vi "Update Control from Metadata.vi"(6 "default_value":variant, 8 "error in":errorcluster, 9 "control name":string, 10 "parameter data":T1[](array[typedef]), 11 "vi refnum":refnum<vi>) -> (0 "error out":errorcluster)   [LabVIEW 2021, in "MeasurementClient Editor.lvlib"]
uses:
  MeasurementClient Editor.lvlib
  <vilib>/gRPC/Generated APIs/ni/measurementlink/measurement/v2/Measurement Service Client V2/RPC Messages/ni_measurementlink_measurement_v2_ConfigurationParameter.ctl
  <vilib>/gRPC/Generated APIs/ni/measurementlink/measurement/v2/Measurement Service Client V2/RPC Messages/google_protobuf_Field_Kind.ctl
  <vilib>/gRPC/Generated APIs/ni/measurementlink/measurement/v2/Measurement Service Client V2/RPC Messages/ni_measurementlink_measurement_v2_ConfigurationParameter_AnnotationsEntry.ctl
  <vilib>/Utility/miscctls.llb/LVPositionTypeDef.ctl
  <vilib>/gRPC/Generated APIs/ni/measurementlink/measurement/v2/Measurement Service Client V2/Measurement Service Client V2.lvlib
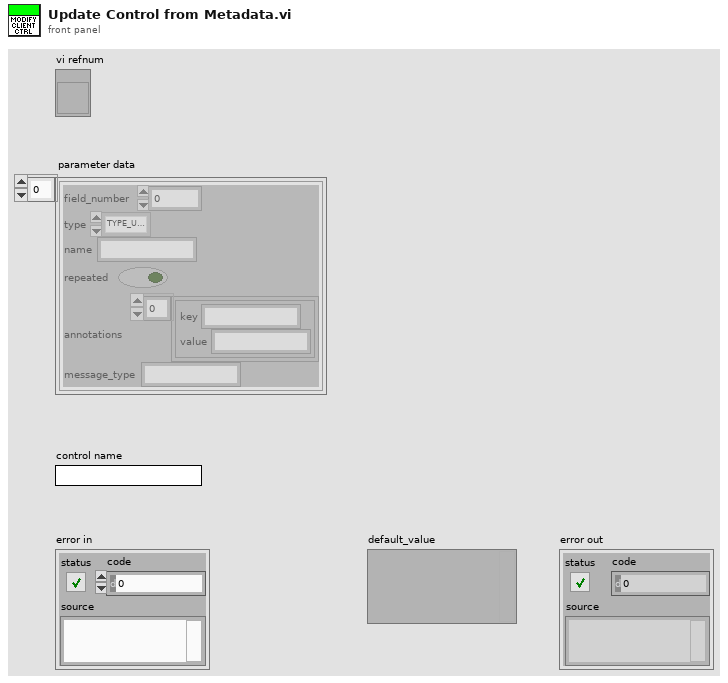
[diagram p1: front panel]
types:
  T1 = typedef "Measurement Service Client V2.lvlib/ni_measurementlink_measurement_v2_ConfigurationParameter.ctl" = cluster{"field_number":i32, "type":T2, "name":string, "repeated":bool, "annotations":T3[], "message_type":string}
  T2 = typedef "Measurement Service Client V2.lvlib/google_protobuf_Field_Kind.ctl" = enum32{"TYPE_UNKNOWN", "TYPE_DOUBLE", "TYPE_FLOAT", "TYPE_INT64", "TYPE_UINT64", "TYPE_INT32", "TYPE_FIXED64", "TYPE_FIXED32", "TYPE_BOOL", "TYPE_STRING", "TYPE_GROUP", "TYPE_MESSAGE", "TYPE_BYTES", "TYPE_UINT32", "TYPE_ENUM", "TYPE_SFIXED32", "TYPE_SFIXED64", "TYPE_SINT32", "TYPE_SINT64"}
  T3 = typedef "Measurement Service Client V2.lvlib/ni_measurementlink_measurement_v2_ConfigurationParameter_AnnotationsEntry.ctl" = cluster{"key":string, "value":string}
  T4 = typedef "LVPositionTypeDef.ctl" = cluster{"Left":i32, "Top":i32}
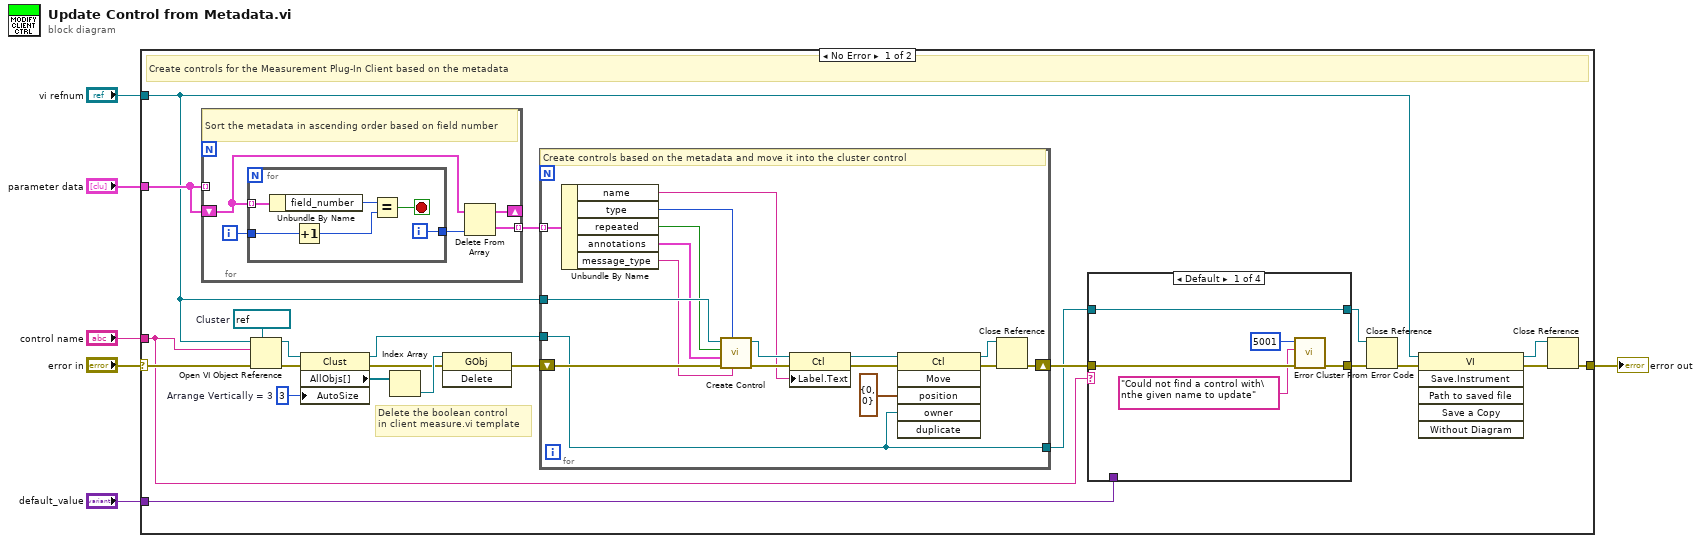
[diagram p0: block diagram]
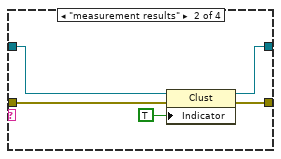
[diagram p2: hidden frame]
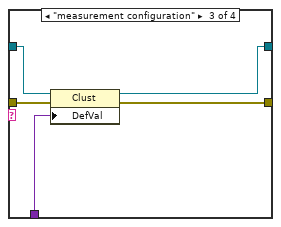
[diagram p3: hidden frame]
diagram:
  n1 = case shown="No Error" "error in" {
    selector: "error in" -> [w23 w75]
    tunnel: "control name" -> [w15 _]
    tunnel: "parameter data" -> [w13 _]
    tunnel: "vi refnum" -> [w10 _]
    tunnel: [w8 w75] -> w3
    tunnel: "default_value" -> [w7 _]
    frame No Error {
      w22 = u32 3  # Arrange Vertically = 3
      w29 = refnum<vi> refnum  # Cluster
      # "Delete the boolean control\nin client measure.vi template"
      # "Create controls for the Measurement Plug-In Client based on the metadata"
      n2 = for {
        shift-right: [w48] -> _
        shift-left: w13 -> [w49]
        tunnel: [w47] -> w14 mode=indexing
        tunnel: w13 -> [_] mode=indexing
        i -> [w51]
        # "Sort the metadata in ascending order based on field number"
        n3 = for {
          tunnel: w49 -> [w54] mode=indexing
          tunnel: w51 -> [w57]
          tunnel: [w53] -> w50
          i -> [w53]
          stop <- w52 stop-if-true
          n4 = Unbundle By Name(w54) -> ("field_number"=w56:i32)
          n5 = Increment(x=w57) -> (x+1=w55:i32)
          n6 = Equal?(x=w56, y=w55) -> (x = y?=w52:bool)
        }
        n7 = Delete From Array(array=w49, index=w50) -> (deleted portion=w47:T1, array with subset deleted=w48:T1[])  [unwired: 1 in]
      }
      n8 = Open VI Object Reference(7:w29, 8:w23, 10:w15, 11:w10) -> (0:w27:errorcluster, 3:w28:refnum<vi>)
      n9 = property class="Clust"(reference=w28, error in=w27, "AutoSize"=w22) -> (reference out=w19:refnum<vi>, error out=w24:errorcluster, "AllObjs[]"=w26:refnum<vi>[])
      n10 = Index Array(array=w26) -> (element=w25:refnum<vi>)  [unwired: 1 in]
      n11 = invoke class="GObj" method="Delete"(reference=w25, error in=w24) -> (error out=w21:errorcluster)  [unwired: 1 in, 2 out]
      n12 = for {
        shift-right: [w34] -> w20
        shift-left: w21 -> [w46]
        tunnel: w10 -> [w44]
        tunnel: w19 -> [w32]
        tunnel: [w32] -> w17
        tunnel: w14 -> [w30] mode=indexing
        # "Create controls based on the metadata and move it into the cluster control"
        n13 = Unbundle By Name(w30) -> ("name"=w38:string, "type"=w42:T2, "repeated"=w43:bool, "annotations"=w41:T3[], "message_type"=w40:string)
        n14 = call "Create Control.vi"("message_type"=w40, "type"=w42, "error in"=w46, "annotations"=w41, "is repeated?"=w43, "vi refnum"=w44) -> ("error out"=w45:errorcluster, "control ref"=w39:refnum<vi>)  [unwired: 4 in]
        n15 = property class="Ctl"(reference=w39, error in=w45, "Label.Text"=w38) -> (reference out=w37:refnum<vi>, error out=w36:errorcluster)
        n16 = invoke class="Ctl" method="Move"(reference=w37, error in=w36, "position"=T4 {"Left"=0, "Top"=0}, "owner"=w32) -> (reference out=w33:refnum<vi>, error out=w35:errorcluster)  [unwired: 2 in, 4 out]
        n17 = Close Reference(reference=w33, error in (no error)=w35) -> (error out=w34:errorcluster)
      }
      n18 = case shown="Default" w15 {
        tunnel: w20 -> [w62 w67 w72 w73]
        tunnel: [w60 w66 w71 w73] -> w18
        tunnel: w17 -> [w61 w65 w70 w74]
        tunnel: [w61 w64 w69 w74] -> w16
        tunnel: w7 -> [_ _ w68 _]
        frame Default {
          n19 = call <vilib>:"Error Cluster From Error Code.vi"("error in (no error)"=w62, "error message (\"\")"="Could not find a control with\nthe given name to update" ("error message (\"\")"), "error code (0)"=5001) -> ("error out"=w60:errorcluster)  [unwired: 6 in]
        }
        frame "measurement results" {
          n20 = property class="Clust"(reference=w65, error in=w67, "Indicator"=TRUE) -> (reference out=w64:refnum<vi>, error out=w66:errorcluster)
        }
        frame "measurement configuration" {
          n21 = property class="Clust"(reference=w70, error in=w72, "DefVal"=w68) -> (reference out=w69:refnum<vi>, error out=w71:errorcluster)
        }
        frame "configuration" {
        }
      }
      n22 = Close Reference(reference=w16, error in (no error)=w18) -> (error out=w9:errorcluster)
      n23 = invoke class="VI" method="Save.Instrument"(reference=w10, error in=w9) -> (reference out=w12:refnum<vi>, error out=w11:errorcluster)  [unwired: 4 in, 4 out]
      n24 = Close Reference(reference=w12, error in (no error)=w11) -> (error out=w8:errorcluster)
    }
    frame Error {
      # "Pass"
    }
  }
  "error out" <- w3
